vi "hysteresis.vi"() -> ()   [LabVIEW 2014]
panel:
  out "Result 2":bool
  in  "Threshold Stop 1":dbl
  out "Result 1":bool
  out "slide":dbl
  in  "Offset":dbl
  in  "Threshold Start":dbl
  in  "Slide":dbl(slide) scale=0.0..10.0
  out "?":bool=TRUE
  in  "stop":bool
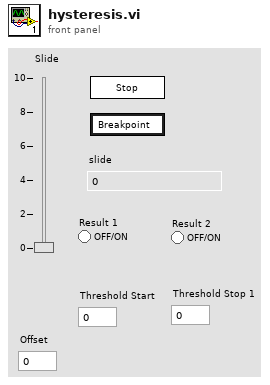
[diagram p1: front panel]
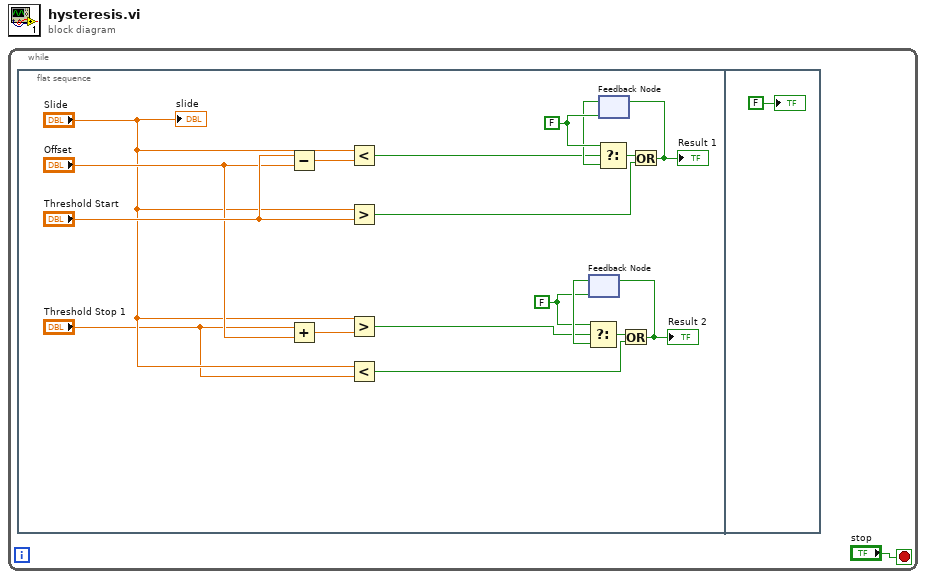
[diagram p0: block diagram]
diagram:
  n1 = while {
    stop <- "stop" stop-if-true
    n2 = flat-sequence {
      frame #0 {
        w4 = FALSE
        w17 = FALSE
        n3 = Subtract(x="Threshold Start", y="Offset") -> (x-y=w19:dbl)
        n4 = Add(x="Threshold Stop 1", y="Offset") -> (x+y=w11:dbl)
        n5 = Less?(x="Slide", y=w19) -> (x < y?=w15:bool)
        n6 = Greater?(x="Slide", y="Threshold Start") -> (0:w13:bool)
        n7 = Greater?(x="Slide", y=w11) -> (0:w2:bool)
        n8 = Less?(x="Slide", y="Threshold Stop 1") -> (x < y?=w3:bool)
        n9 = feedback #1(w4) -> (w5:bool)
        n10 = Select(t=w4, s=w2, f=w5) -> (s? t:f=w6:bool)
        n11 = feedback #2(w17) -> (w16:bool)
        n12 = Select(t=w17, s=w15, f=w16) -> (s? t:f=w14:bool)
        n13 = Or(x=w6, y=w3) -> (x .or. y?=w7:bool)
        "Result 2" <- w7
        n14 = feedback-in #1(w7) -> ()
        n15 = Or(x=w14, y=w13) -> (x .or. y?=w12:bool)
        "Result 1" <- w12
        n16 = feedback-in #2(w12) -> ()
        "slide" <- "Slide"
      }
      frame #1 {
        "?" <- FALSE
      }
    }
  }
